vi "Cell Space_Table.vi"(4 "Row Header in":string[](array[string]), 6 "Col Header in":string[](array[string]), 7 "빈내용 숨기기?(F)":bool, 8 "error in":errorcluster caption="에러 입력(에러 없음)", 10 "Data in":string[][](array[string]), 11 "테이블 참조 in":refnum<vi>) -> (0 "error out":errorcluster caption="에러 출력", 1 "열(U32)":u32, 3 "테이블 참조 Out":refnum<vi>)   [LabVIEW 2020]
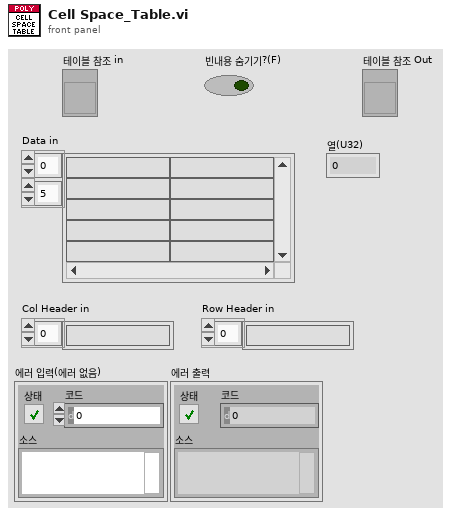
[diagram p1: front panel]
types:
  T1 = cluster{"left":i16, "top":i16, "right":i16, "bottom":i16}
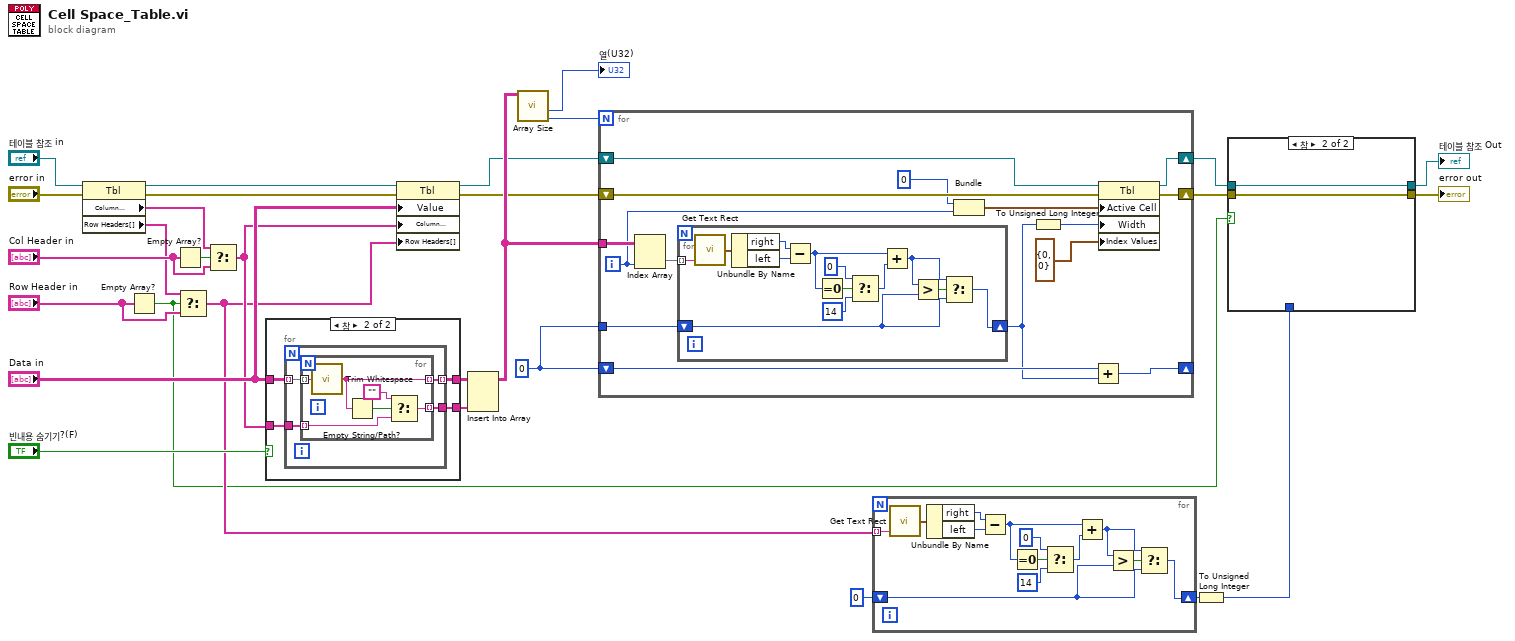
[diagram p0: block diagram]
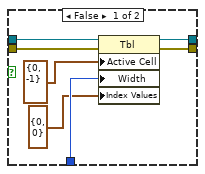
[diagram p2: hidden frame]
diagram:
  w29 = i16 0 ("인덱스")
  n1 = property on="프로퍼티 노드" class="Tbl"(reference="테이블 참조 in", error in="error in") -> (reference out=w14:refnum<vi>, error out=w16:errorcluster, "Column Headers[]"=w13:string[], "Row Headers[]"=w12:string[])
  n2 = Empty Array?(array="Row Header in") -> (empty?=w3:bool)
  n3 = Empty Array?(array="Col Header in") -> (empty?=w20:bool)
  n4 = Select(t=w12, s=w3, f="Row Header in") -> (s? t:f=w9:string[])
  n5 = Select(t=w13, s=w20, f="Col Header in") -> (s? t:f=w18:string[])
  n6 = case shown="참" "빈내용 숨기기?(F)" {
    tunnel: "Data in" -> [w31 w35]
    tunnel: [w31 w34] -> w27
    tunnel: w18 -> [w30 w33]
    tunnel: [w30 w32] -> w26
    frame False {
    }
    frame True {
      n7 = for {
        tunnel: w35 -> [w39] mode=indexing
        tunnel: [w38] -> w34 mode=indexing
        tunnel: w33 -> [w37]
        tunnel: [w36] -> w32
        n8 = for {
          tunnel: w39 -> [w45] mode=indexing
          tunnel: [w44] -> w38 mode=indexing
          tunnel: w37 -> [w42] mode=indexing
          tunnel: [w41] -> w36 mode=indexing
          n9 = call <vilib>:"Trim Whitespace.vi"("string"=w45) -> ("trimmed string"=w44:string)  [unwired: 1 in]
          n10 = Empty String/Path?(string/path=w44) -> (empty?=w43:bool)
          n11 = Select(t="", s=w43, f=w42) -> (s? t:f=w41:string)
        }
      }
    }
  }
  n12 = property on="프로퍼티 노드" class="Tbl"(reference=w14, error in=w16, "Value"="Data in", "Column Headers[]"=w18, "Row Headers[]"=w9) -> (reference out=w22:refnum<vi>, error out=w24:errorcluster)
  n13 = Insert Into Array(array=w27, new element=w26) -> (w28:string[][])  [unwired: 2 in]
  n14 = call "Array Size.vi"("Data in"=w28) -> ("열(I32)"=w2:i32, "열(U32)"=→"열(U32)":u32)  [unwired: 7 in, 2 out]
  n15 = for {
    N: w2 -> [_]
    shift-right: [w59] -> w5
    shift-left: w24 -> [w60]
    tunnel: w28 -> [w58]
    shift-right: [w52] -> _
    shift-left: w29 -> [w51]
    shift-right: [w49] -> w8
    shift-left: w22 -> [w53]
    tunnel: w29 -> [w48]
    i -> [w56]
    n16 = Index Array(array=w58, index (col)=w56) -> (element=w57:string[])  [unwired: 1 in]
    n17 = for {
      tunnel: w57 -> [w70] mode=indexing
      shift-right: [w71] -> w50
      shift-left: w48 -> [w72]
      n18 = call <vilib>:"Get Text Rect.vi"("text"=w70) -> ("rect"=w69:T1)  [unwired: 8 in]
      n19 = Unbundle By Name(w69) -> ("right"=w68:i16, "left"=w67:i16)
      n20 = Subtract(x=w68, y=w67) -> (x-y=w65:i16)
      n21 = Equal To 0?(x=w65) -> (x = 0?=w64:bool)
      n22 = Select(t=i16 0 ("y"), s=w64, f=i16 14 ("y")) -> (s? t:f=w61:i16)
      n23 = Add(x=w65, y=w61) -> (x+y=w66:i16)
      n24 = Greater?(x=w66, y=w72) -> (0:w73:bool)
      n25 = Select(t=w66, s=w73, f=w72) -> (s? t:f=w71:i16)
    }
    n26 = Bundle("인덱스"=0, w56) -> (w54:cluster{"인덱스":i32, i32})  [unwired: 1 in]
    n27 = To Unsigned Long Integer(number=w50) -> (unsigned 32bit integer=w47:u32)
    n28 = Add(x=w51, y=w50) -> (x+y=w52:i16)
    n29 = property on="프로퍼티 노드" class="Tbl"(reference=w53, error in=w60, "Active Cell"=w54, "Width"=w47, "Index Values"=cluster{i32, i32} {0, 0}) -> (reference out=w49:refnum<vi>, error out=w59:errorcluster)
  }
  n30 = for {
    tunnel: w9 -> [w83] mode=indexing
    shift-right: [w84] -> w11
    shift-left: i16 0 ("인덱스") -> [w85]
    n31 = call <vilib>:"Get Text Rect.vi"("text"=w83) -> ("rect"=w82:T1)  [unwired: 8 in]
    n32 = Unbundle By Name(w82) -> ("right"=w81:i16, "left"=w80:i16)
    n33 = Subtract(x=w81, y=w80) -> (x-y=w78:i16)
    n34 = Equal To 0?(x=w78) -> (x = 0?=w77:bool)
    n35 = Select(t=i16 0 ("y"), s=w77, f=i16 14 ("y")) -> (s? t:f=w74:i16)
    n36 = Add(x=w78, y=w74) -> (x+y=w79:i16)
    n37 = Greater?(x=w79, y=w85) -> (0:w86:bool)
    n38 = Select(t=w79, s=w86, f=w85) -> (s? t:f=w84:i16)
  }
  n39 = To Unsigned Long Integer(number=w11) -> (unsigned 32bit integer=w10:u32)
  n40 = case shown="참" w3 {
    tunnel: w10 -> [w93 _]
    tunnel: w8 -> [w91 w94]
    tunnel: [w90 w94] -> w7
    tunnel: [w89 w95] -> w6
    tunnel: w5 -> [w88 w95]
    frame False {
      n41 = property on="프로퍼티 노드" class="Tbl"(reference=w91, error in=w88, "Active Cell"=cluster{i32, i32} {0, -1}, "Width"=w93, "Index Values"=cluster{i32, i32} {0, 0}) -> (reference out=w90:refnum<vi>, error out=w89:errorcluster)
    }
    frame True {
    }
  }
  "테이블 참조 Out" <- w7
  "error out" <- w6
